vi "ClusterToStringArray.vi"(11 "cluster":T1={"SI camera info"={"Observer Name"="", "object name"="", "File name base"="", "Camera Color"="Red", "Exp type tab"=enum."Object", "Number of Exp"=1.0, "Exp time"=0.0, "CCD Readout Speed"=5, "CCD ROI Mode"=10, "Hg(Ar)"=FALSE, "Cu"=FALSE, "Ne"=FALSE, "Bulb"=FALSE, "Ar"=FALSE, "Quartz"=FALSE, "Quartz Percent"=0.0, "Fe"=FALSE, "Notes"="", "Target Number"="", "Dome Percent"=0.0, "Dome"=FALSE}, "Configuration"={"Primary Filter"="<NO FILTER>", "Secondary Filter"="<NO FILTER>", "Slit Mask"="<NO MASK>", "Grating"="<NO GRATING>", "CS Target"=0.0, "GS Target"=0.0, "Coll Focus"=1000, "Camera Focus"=0, "Name"="", "User"="", "Date"="", "Comment"="", "use Flexure Comp?"=FALSE, "Select Mode:"=0}, "Path to Configuration File"=path ""} {"Configuration"."Select Mode:" items=["Custom", "Imaging", "300 All", "600 UV", "600 Blue", "600 Mid", "600 Red", "1200 m0", "1200 m1", "1200 m2", "1200 m3", "1200 m4", "1200 m5", "1200 m6", "1200 m7", "1200 RESOLVE", "400 m1", "400 m2", "930 m1", "930 m2", "930 m3", "930 m4", "930 m5", "930 m6", "400WD", "930TP", "400Fermi", "400Padgett", "400Lewis", "400Crotts", "600BLee", "600RLee", "400WW"]; "SI camera info"."Dome Percent" min=0.0 step=1.0; "SI camera info"."Quartz Percent" min=0.0 step=1.0; "SI camera info"."CCD Readout Speed" items=["750 kHz, ATTN 0", "750 kHz, ATTN 2", "344 kHz, ATTN 0", "344 kHz, ATTN 3", "100 kHz, ATTN 2", "100 kHz, ATTN 3"]; "SI camera info"."CCD ROI Mode" items=["Imaging, 1x1  "=0, "Imaging, 2x2"=1, "Imaging, 3x3"=2, "Spectroscopic, 1x1"=3, "Spectroscopic, 2x2"=4, "Spectroscopic, 3x3"=5, "MOS, 1x1"=11, "MOS, 2x2"=12, "MOS, 3x3"=13, "Slicer"=6, "Spectroscopic, ZZ Ceti"=14, "Slit Imaging/Alignment"=7, "MOS Imaging/Alignment"=10, "Set user-defined ROI..."=21, "Custom Mode"=9]; "SI camera info"."Number of Exp" min=0.0 step=0.5; "SI camera info"."Exp time" min=0.0 step=0.1}) -> (3 "Array":string[](array[string]))   [LabVIEW 2015]
panel:
  in  "Steps":dbl
  in  "Delta":dbl
  in  "Start":dbl
  # "Or"
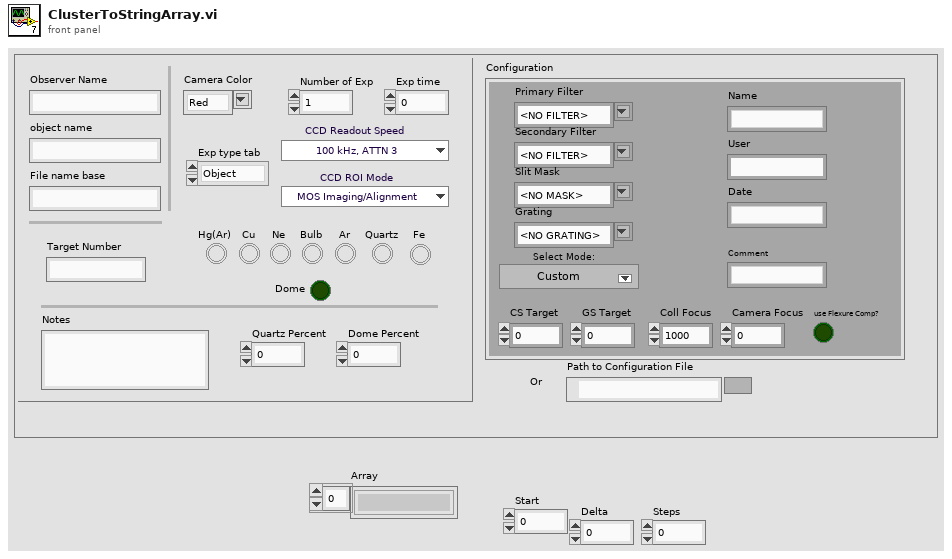
[diagram p1: front panel]
types:
  T1 = cluster{"SI camera info":cluster{"Observer Name":string, "object name":string, "File name base":string, "Camera Color":string, "Exp type tab":enum16{"Object", "Flat", "Comp", "Dark", "Zero"}, "Number of Exp":dbl, "Exp time":dbl, "CCD Readout Speed":u8, "CCD ROI Mode":u16, "Hg(Ar)":bool, "Cu":bool, "Ne":bool, "Bulb":bool, "Ar":bool, "Quartz":bool, "Quartz Percent":dbl, "Fe":bool, "Notes":string, "Target Number":string, "Dome Percent":dbl, "Dome":bool}, "Configuration":cluster{"Primary Filter":string, "Secondary Filter":string, "Slit Mask":string, "Grating":string, "CS Target":dbl, "GS Target":dbl, "Coll Focus":i32, "Camera Focus":i32, "Name":string, "User":string, "Date":string, "Comment":string, "use Flexure Comp?":bool, "Select Mode:":u16}, "Path to Configuration File":path}
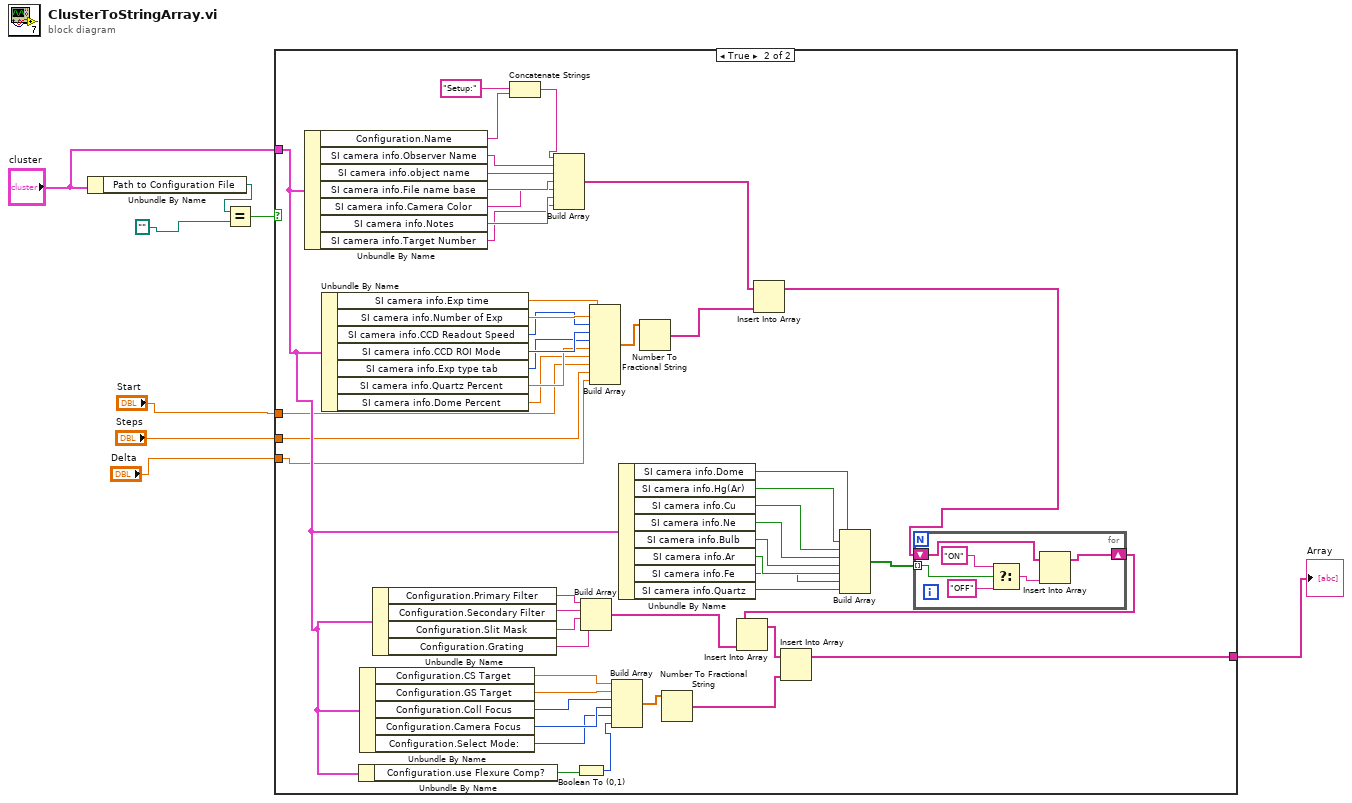
[diagram p0: block diagram]
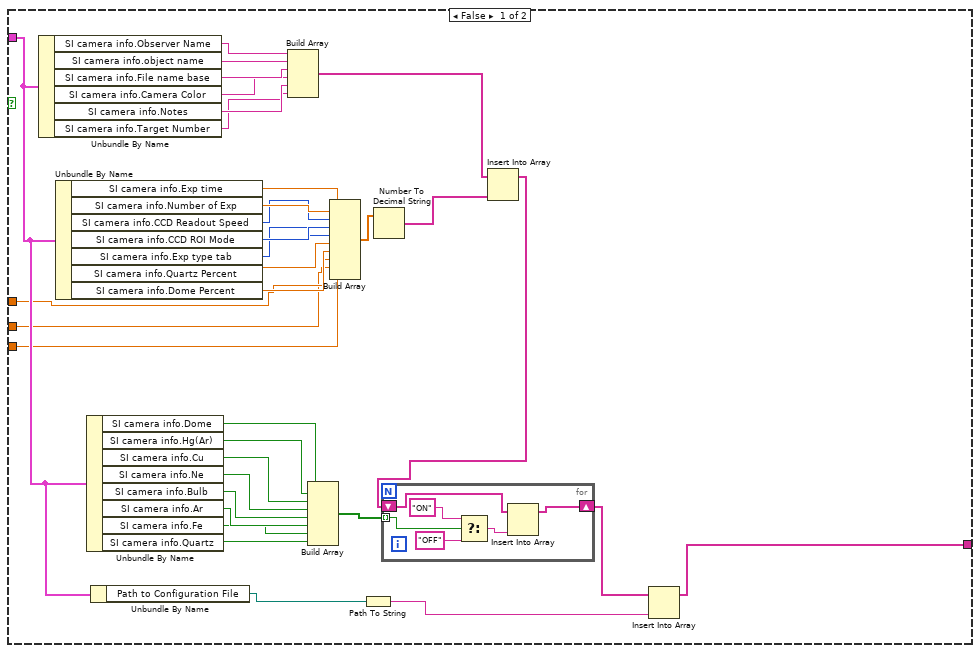
[diagram p2: hidden frame]
diagram:
  n1 = Unbundle By Name("cluster") -> ("Path to Configuration File"=w8:path)
  n2 = Equal?(x=w8, y=path "") -> (x = y?=w7:bool)
  n3 = case shown="True" w7 {
    tunnel: "cluster" -> [w42 w73]
    tunnel: [w14 w57] -> w5
    tunnel: "Start" -> [w12 w51]
    tunnel: "Steps" -> [w11 w52]
    tunnel: "Delta" -> [w10 w53]
    frame False {
      n4 = Unbundle By Name(w42) -> ("SI camera info.Observer Name"=w33:string, "SI camera info.object name"=w32:string, "SI camera info.File name base"=w31:string, "SI camera info.Camera Color"=w30:string, "SI camera info.Notes"=w29:string, "SI camera info.Target Number"=w28:string)
      n5 = Unbundle By Name(w42) -> ("SI camera info.Exp time"=w27:dbl, "SI camera info.Number of Exp"=w26:dbl, "SI camera info.CCD Readout Speed"=w25:u8, "SI camera info.CCD ROI Mode"=w24:u16, "SI camera info.Exp type tab"=w23:enum16{"Object", "Flat", "Comp", "Dark", "Zero"}, "SI camera info.Quartz Percent"=w22:dbl, "SI camera info.Dome Percent"=w13:dbl)
      n6 = Unbundle By Name(w42) -> ("SI camera info.Dome"=w9:bool, "SI camera info.Hg(Ar)"=w40:bool, "SI camera info.Cu"=w39:bool, "SI camera info.Ne"=w38:bool, "SI camera info.Bulb"=w37:bool, "SI camera info.Ar"=w36:bool, "SI camera info.Fe"=w35:bool, "SI camera info.Quartz"=w34:bool)
      n7 = Unbundle By Name(w42) -> ("Path to Configuration File"=w16:path)
      n8 = Build Array(w33, w32, w31, w30, w29, w28) -> (w19:string[])
      n9 = Build Array(w9, w40, w39, w38, w37, w36, w35, w34) -> (w41:bool[])
      n10 = Build Array(w27, w26, w25, w24, w23, w22, w13, w12, w11, w10) -> (w21:dbl[])
      n11 = Path To String(path=w16) -> (string=w15:string)
      n12 = Number To Decimal String(number=w21) -> (decimal integer string=w20:string[])  [unwired: 1 in]
      n13 = Insert Into Array(array=w19, new element=w20) -> (w18:string[])  [unwired: 1 in]
      n14 = for {
        tunnel: w41 -> [w48] mode=indexing
        shift-right: [w43] -> w17
        shift-left: w18 -> [w44]
        n15 = Select(t="ON", s=w48, f="OFF") -> (s? t:f=w45:string)
        n16 = Insert Into Array(array=w44, new element=w45) -> (w43:string[])  [unwired: 1 in]
      }
      n17 = Insert Into Array(array=w17, new element=w15) -> (w14:string[])  [unwired: 1 in]
    }
    frame True {
      n18 = Unbundle By Name(w73) -> ("Configuration.Name"=w56:string, "SI camera info.Observer Name"=w90:string, "SI camera info.object name"=w89:string, "SI camera info.File name base"=w88:string, "SI camera info.Camera Color"=w87:string, "SI camera info.Notes"=w86:string, "SI camera info.Target Number"=w85:string)
      n19 = Unbundle By Name(w73) -> ("SI camera info.Exp time"=w84:dbl, "SI camera info.Number of Exp"=w83:dbl, "SI camera info.CCD Readout Speed"=w82:u8, "SI camera info.CCD ROI Mode"=w81:u16, "SI camera info.Exp type tab"=w80:enum16{"Object", "Flat", "Comp", "Dark", "Zero"}, "SI camera info.Quartz Percent"=w79:dbl, "SI camera info.Dome Percent"=w50:dbl)
      n20 = Unbundle By Name(w73) -> ("Configuration.use Flexure Comp?"=w61:bool)
      n21 = Unbundle By Name(w73) -> ("Configuration.CS Target"=w66:dbl, "Configuration.GS Target"=w65:dbl, "Configuration.Coll Focus"=w64:i32, "Configuration.Camera Focus"=w63:i32, "Configuration.Select Mode:"=w62:u16)
      n22 = Unbundle By Name(w73) -> ("Configuration.Primary Filter"=w72:string, "Configuration.Secondary Filter"=w71:string, "Configuration.Slit Mask"=w70:string, "Configuration.Grating"=w69:string)
      n23 = Concatenate Strings("Setup:", w56) -> (w54:string)
      n24 = Build Array(w54, w90, w89, w88, w87, w86, w85) -> (w76:string[])
      n25 = Boolean To (0,1)(Boolean=w61) -> (0, 1=w60:i16)
      n26 = Build Array(w72, w71, w70, w69) -> (w68:string[])
      n27 = Build Array(w84, w83, w82, w81, w80, w79, w50, w51, w52, w53) -> (w78:dbl[])
      n28 = Build Array(w66, w65, w64, w63, w62, w60) -> (w67:dbl[])
      n29 = Unbundle By Name(w73) -> ("SI camera info.Dome"=w49:bool, "SI camera info.Hg(Ar)"=w97:bool, "SI camera info.Cu"=w96:bool, "SI camera info.Ne"=w95:bool, "SI camera info.Bulb"=w94:bool, "SI camera info.Ar"=w93:bool, "SI camera info.Fe"=w92:bool, "SI camera info.Quartz"=w91:bool)
      n30 = Number To Fractional String(number=w78) -> (F-format string=w77:string[])  [unwired: 3 in]
      n31 = Number To Fractional String(number=w67) -> (F-format string=w58:string[])  [unwired: 3 in]
      n32 = Insert Into Array(array=w76, new element=w77) -> (w75:string[])  [unwired: 1 in]
      n33 = Build Array(w49, w97, w96, w95, w94, w93, w92, w91) -> (w98:bool[])
      n34 = for {
        tunnel: w98 -> [w104] mode=indexing
        shift-right: [w99] -> w74
        shift-left: w75 -> [w100]
        n35 = Select(t="ON", s=w104, f="OFF") -> (s? t:f=w101:string)
        n36 = Insert Into Array(array=w100, new element=w101) -> (w99:string[])  [unwired: 1 in]
      }
      n37 = Insert Into Array(array=w74, new element=w68) -> (w59:string[])  [unwired: 1 in]
      n38 = Insert Into Array(array=w59, new element=w58) -> (w57:string[])  [unwired: 1 in]
    }
  }
  "Array" <- w5
